vi "USBClient.vi"() -> ()   [LabVIEW 2018]
uses:
  <vilib>/daq.io/MQTT LabVIEW Client/Controls/User_Info.ctl
  <vilib>/daq.io/MQTT LabVIEW Client/Controls/Connect_Flags.ctl
  <vilib>/daq.io/MQTT LabVIEW Client/Controls/QoS.ctl
  <vilib>/daq.io/MQTT LabVIEW Client/Controls/DUP_Flag.ctl
  <vilib>/daq.io/MQTT LabVIEW Client/Controls/Retain_Flag.ctl
  <vilib>/daq.io/MQTT LabVIEW Client/Controls/Connection_Return_Codes.ctl
  <vilib>/daq.io/MQTT LabVIEW Client/MQTT_Functions.lvlib
panel:
  out "error out":errorcluster
  in  "Stop":bool
  in  "Start":bool
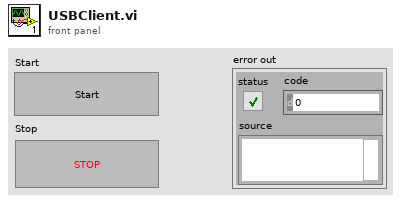
[diagram p1: front panel]
types:
  T1 = typedef "MQTT_Functions.lvlib/QoS.ctl" = enum8{"At most once", "At least once", "Exactly once", "Reserved"}
  T2 = typedef "MQTT_Functions.lvlib/DUP_Flag.ctl" = bool
  T3 = typedef "MQTT_Functions.lvlib/Retain_Flag.ctl" = bool
  T4 = cluster{"QoS":T1, "DUP":T2, "Retain":T3, "Keep Alive (sec)":u16}
  T5 = typedef "MQTT_Functions.lvlib/Connect_Flags.ctl" = cluster{"user name":bool, "password":bool, "will retain":bool, "will flag":bool, "clean session":bool, "reserved":bool, "will QoS":T1}
  T6 = typedef "MQTT_Functions.lvlib/User_Info.ctl" = cluster{"User Name":string, "Password":string}
  T7 = cluster{"Connect Meta":cluster{"QoS":T1, "DUP":T2, "Retain":T3, "Keep Alive (sec)":u16}, "Connect Flags":T5, "MQTT Broker":cluster{"address (IP)":string, "port":u16}, "User Info":T6, "Client ID":string}
  T8 = typedef "MQTT_Functions.lvlib/Connection_Return_Codes.ctl" = enum16{"Connection accepted", "Connection refused: unacceptable protocol version", "Connection refused: identifier rejected", "Connection refused: Server unavailable", "Connection refused: bad user name or password", "Connection refused: not authorized"}
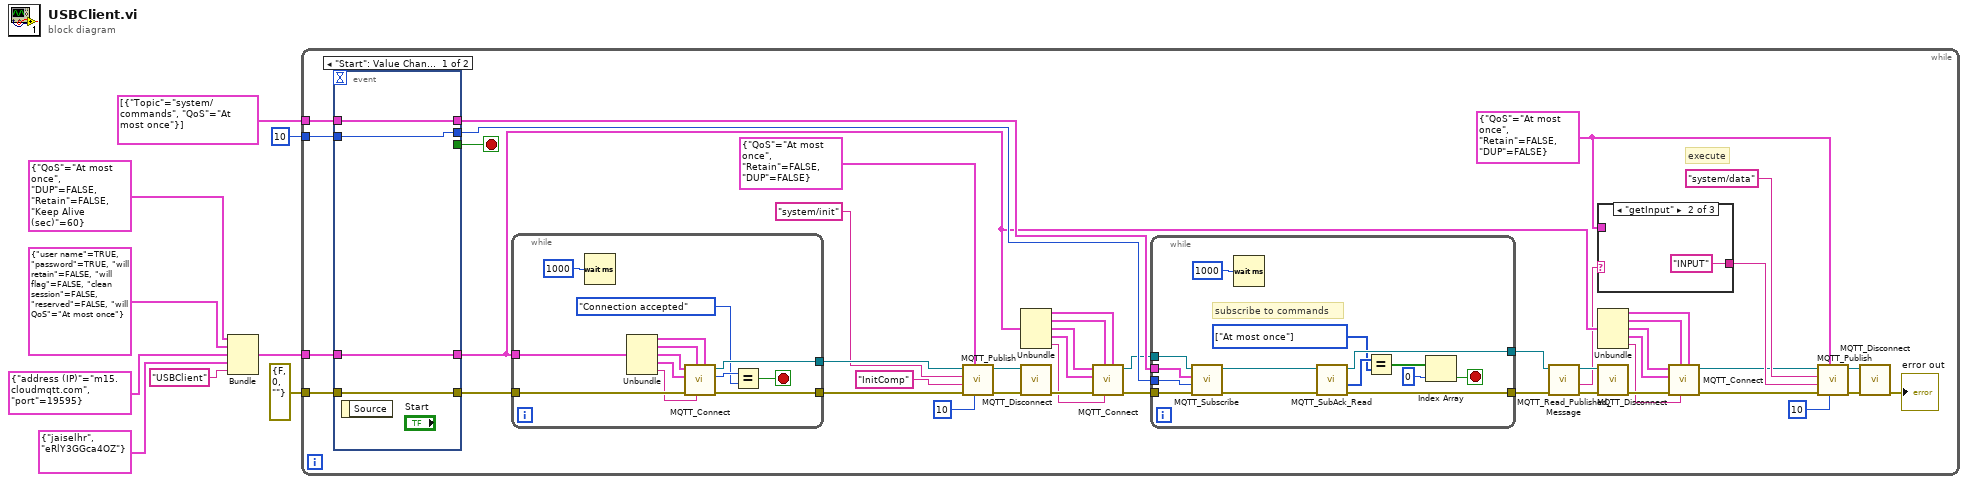
[diagram p0: block diagram]
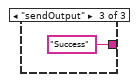
[diagram p3: hidden frame]
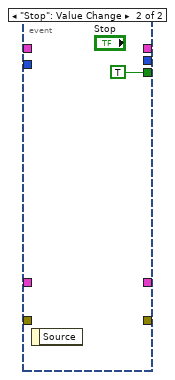
[diagram p4: hidden frame]
diagram:
  n1 = Bundle("Connect Meta"=T4 {"QoS"=enum."At most once", "DUP"=FALSE, "Retain"=FALSE, "Keep Alive (sec)"=60}, "Connect Flags"=T5 {"user name"=TRUE, "password"=TRUE, "will retain"=FALSE, "will flag"=FALSE, "clean session"=FALSE, "reserved"=FALSE, "will QoS"=enum."At most once"}, "MQTT Broker"=cluster{"address (IP)":string, "port":u16} {"address (IP)"="m15.cloudmqtt.com", "port"=19595}, "User Info"=T6 {"User Name"="jaiselhr", "Password"="eRlY3GGca4OZ"}, "Client ID"="USBClient") -> (w1:T7)  [unwired: 1 in]
  n2 = while {
    tunnel: errorcluster {"status"=FALSE, "code"=0, "source"=""} ("error in (no error)") -> [w53]
    tunnel: cluster{"Topic":string, "QoS":T1}[] [{"Topic"="system/commands", "QoS"=enum."At most once"}] ("Subscription Info Array") -> [w51]
    tunnel: u16 10 ("Message ID") -> [w49]
    tunnel: w1 -> [w27]
    stop <- w54 stop-if-true
    w47 = cluster{"QoS":T1, "Retain":T3, "DUP":T2} {"QoS"=enum."At most once", "Retain"=FALSE, "DUP"=FALSE} ("Publish Meta")
    # "execute"
    n3 = event shown="[0] \"Start\": Value Change" {
      selector: _ -> [_ _]
      dyn-events: _ -> [_ _]
      timeout: _ -> [_ _]
      tunnel: [_ TRUE] -> w54
      tunnel: [w87 _] -> w48
      tunnel: w53 -> [w87 _]
      tunnel: [w86 _] -> w52
      tunnel: w51 -> [w86 _]
      tunnel: [w85 _] -> w50
      tunnel: w49 -> [w85 _]
      tunnel: [w84 _] -> w26
      tunnel: w27 -> [w84 _]
      event "Start": Value Change {
        n4 = event-data() -> ()  [unwired: 1 in, 1 out]
      }
      event "Stop": Value Change {
        n5 = event-data() -> ()  [unwired: 1 in, 1 out]
      }
    }
    n6 = while {
      tunnel: w48 -> [w69]
      tunnel: [w68] -> w41
      tunnel: [w67] -> w40
      tunnel: w26 -> [w62]
      stop <- w64 stop-if-true
      n7 = Wait (ms)(milliseconds to wait=u32 1000) -> ()  [unwired: 1 out]
      n8 = Unbundle(w62) -> ("Connect Meta"=w61:T4, "Connect Flags"=w60:T5, "MQTT Broker"=w59:cluster{"address (IP)":string, "port":u16}, "User Info"=w58:T6, "Client ID"=w57:string)
      n9 = call <vilib>:"MQTT_Connect.vi"("Connect Meta"=w61, "Client ID"=w57, "Connect Flags"=w60, "error in (no error)"=w69, "User Info"=w58, "MQTT Broker"=w59) -> ("error out"=w68:errorcluster, "Connection Status"=w66:T8, "connection ID out"=w67:refnum<k5>)  [unwired: 3 in]
      n10 = Equal?(x=w66, y=Connection_Return_Codes."Connection accepted") -> (x = y?=w64:bool)
    }
    n11 = call <vilib>:"MQTT_Publish.vi"("Message ID"=u16 10, "Publish Meta"=cluster{"QoS":T1, "Retain":T3, "DUP":T2} {"QoS"=enum."At most once", "Retain"=FALSE, "DUP"=FALSE}, "error in (no error)"=w41, "Message to be published"="InitComp", "Topic"="system/init", "connection ID"=w40) -> ("error out"=w35:errorcluster, "connection ID out"=w34:refnum<k5>)  [unwired: 4 in]
    n12 = Unbundle(w26) -> ("Connect Meta"=w25:T4, "Connect Flags"=w24:T5, "MQTT Broker"=w23:cluster{"address (IP)":string, "port":u16}, "User Info"=w22:T6, "Client ID"=w21:string)
    n13 = call <vilib>:"MQTT_Disconnect.vi"("error in (no error)"=w35, "connection ID"=w34) -> ("error out"=w33:errorcluster)  [unwired: 9 in]
    n14 = call <vilib>:"MQTT_Connect.vi"("Connect Meta"=w25, "Client ID"=w21, "Connect Flags"=w24, "error in (no error)"=w33, "User Info"=w22, "MQTT Broker"=w23) -> ("error out"=w31:errorcluster, "connection ID out"=w32:refnum<k5>)  [unwired: 3 in, 1 out]
    n15 = while {
      tunnel: w32 -> [w83]
      tunnel: w31 -> [w82]
      tunnel: w52 -> [w79]
      tunnel: w50 -> [w78]
      tunnel: [w77] -> w14
      tunnel: [w76] -> w15
      stop <- w71 stop-if-true
      w74 = T1[] [enum."At most once"] items=["At most once", "At least once", "Exactly once", "Reserved"] ("y")
      # "subscribe to commands"
      n16 = call <vilib>:"MQTT_Subscribe.vi"("error in (no error)"=w82, "Message ID"=w78, "Subscription Info Array"=w79, "connection ID"=w83) -> ("error out"=w80:errorcluster, "connection ID out"=w81:refnum<k5>)  [unwired: 6 in]
      n17 = Wait (ms)(milliseconds to wait=u32 1000) -> ()  [unwired: 1 out]
      n18 = call <vilib>:"MQTT_SubAck_Read.vi"("error in (no error)"=w80, "connection ID"=w81) -> ("error out"=w76:errorcluster, "Granted QoS Levels"=w75:T1[], "connection ID out"=w77:refnum<k5>)  [unwired: 7 in]
      n19 = Equal?(x=w75, y=w74) -> (x = y?=w73:bool[])
      n20 = Index Array(array=w73, index=0) -> (element=w71:bool)
    }
    n21 = call <vilib>:"MQTT_Read_Published_Message.vi"("error in (no error)"=w15, "connection ID"=w14) -> ("error out"=w12:errorcluster, "Message"=w11:string, "connection ID out"=w13:refnum<k5>)  [unwired: 4 in, 3 out]
    n22 = case shown="\"getInput\"" w11 {
      tunnel: w47 -> [_ _ _]
      tunnel: [_ "INPUT" ("Message to be published") "Success" ("Message to be published")] -> w45
      frame "False", Default {
      }
      frame "getInput" {
      }
      frame "sendOutput" {
      }
    }
    n23 = Unbundle(w26) -> ("Connect Meta"=w20:T4, "Connect Flags"=w19:T5, "MQTT Broker"=w18:cluster{"address (IP)":string, "port":u16}, "User Info"=w17:T6, "Client ID"=w16:string)
    n24 = call <vilib>:"MQTT_Disconnect.vi"("error in (no error)"=w12, "connection ID"=w13) -> ("error out"=w28:errorcluster)  [unwired: 9 in]
    n25 = call <vilib>:"MQTT_Connect.vi"("Connect Meta"=w20, "Client ID"=w16, "Connect Flags"=w19, "error in (no error)"=w28, "User Info"=w17, "MQTT Broker"=w18) -> ("error out"=w29:errorcluster, "connection ID out"=w30:refnum<k5>)  [unwired: 3 in, 1 out]
    n26 = call <vilib>:"MQTT_Publish.vi"("Message ID"=u16 10, "Publish Meta"=w47, "error in (no error)"=w29, "Message to be published"=w45, "Topic"="system/data", "connection ID"=w30) -> ("error out"=w43:errorcluster, "connection ID out"=w42:refnum<k5>)  [unwired: 4 in]
    n27 = call <vilib>:"MQTT_Disconnect.vi"("error in (no error)"=w43, "connection ID"=w42) -> ("error out"=→"error out":errorcluster)  [unwired: 9 in]
  }
